vi "Quick Usb Open.vi"(8 "error in (no error)":errorcluster, 10 "deviceName":string, 11 "hDevice":u32) -> (0 "error out":errorcluster, 1 "function return":i32, 2 "deviceName out":string, 3 "hDevice out":u32)   [LabVIEW 2011, in "QuickUSB.lvlib"]
doc: "QUSBLIB QRETURN QuickUsbOpen(\n PQHANDLE hDevice, \n PQCHAR deviceName\n);"
uses:
  QuickUSB.lvlib
  QuickUSB.dll
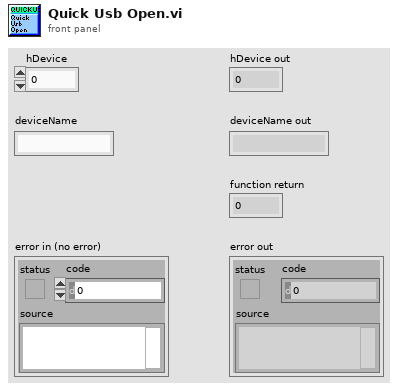
[diagram p1: front panel]
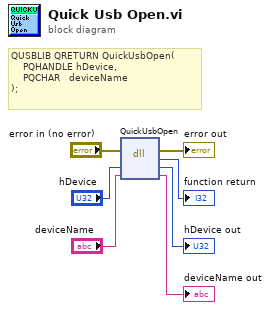
[diagram p0: block diagram]
diagram:
  # "QUSBLIB QRETURN QuickUsbOpen(\n    PQHANDLE hDevice, \n    PQCHAR   deviceName\n);"
  n1 = dll-call lib="C:/QuickUSB/QuickUSB.*" fn="QuickUsbOpen"(error in="error in (no error)", "hDevice"="hDevice", "deviceName"="deviceName") -> (error out=→"error out":errorcluster, →"function return":i32, "hDevice"=→"hDevice out":u32, "deviceName"=→"deviceName out":string)  [unwired: 2 in, 1 out]
